vi "Add Array of New Shared Variables.vi"(7 "Data Type (Variant)":variant, 8 "error in":errorcluster, 9 "Variable Names":string[](array[string]), 10 "Library Path":path, 11 "Selected Library In":refnum<vi>) -> (0 "error out":errorcluster, 3 "Selected Library Out":refnum<vi>)   [LabVIEW 2017, in "Shared Variables Library.lvlib"]
doc: "Adds an array of shared variables, to the selected library."
uses:
  Shared Variables Library.lvlib
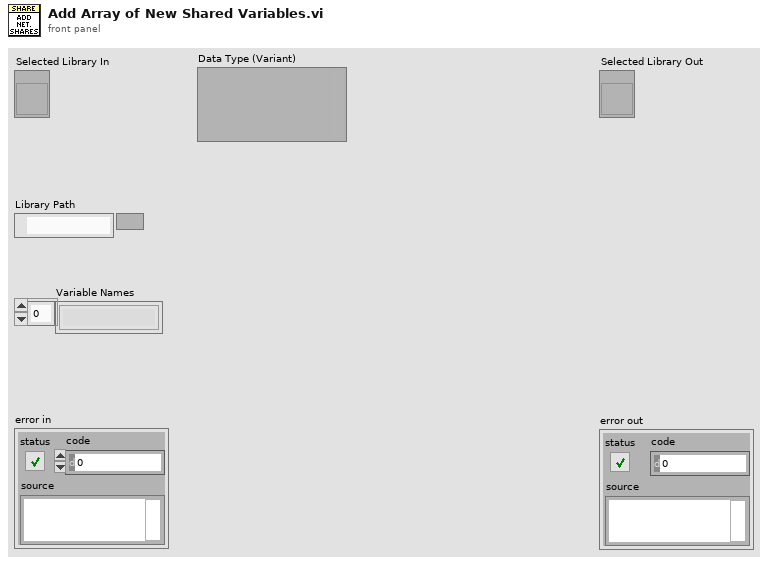
[diagram p1: front panel]
types:
  T1 = enum16{"Single-Process", "Network-Published", "Time-Triggered", "Industrial"}
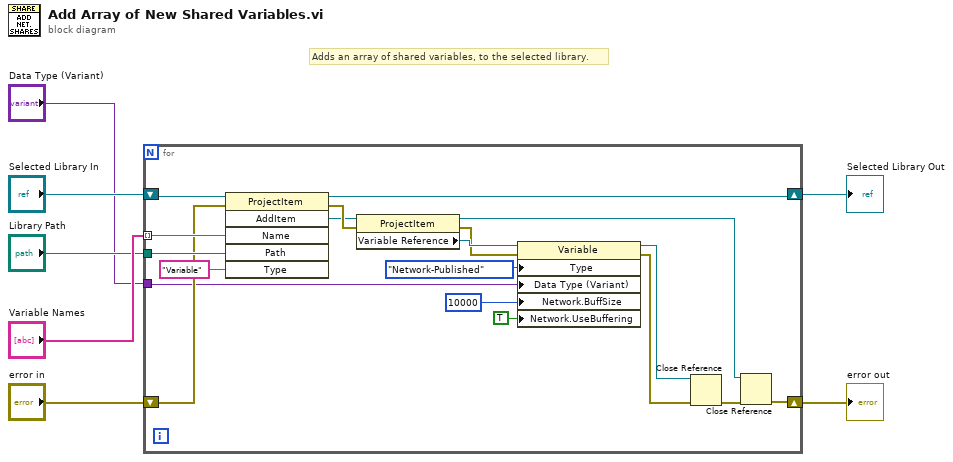
[diagram p0: block diagram]
diagram:
  # "Adds an array of shared variables, to the selected library."
  n1 = for {
    tunnel: "Variable Names" -> [w26] mode=indexing
    tunnel: "Library Path" -> [w23]
    shift-right: [w11] -> w3
    shift-left: "Selected Library In" -> [w24]
    shift-right: [w13] -> w2
    shift-left: "error in" -> [w19]
    tunnel: "Data Type (Variant)" -> [w10]
    n2 = invoke class="ProjectItem" method="AddItem"(reference=w24, error in=w19, "Name"=w26, "Path"=w23, "Type"="Variable") -> (reference out=w11:refnum<vi>, error out=w18:errorcluster, "AddItem"=w15:refnum<vi>)  [unwired: 1 in, 3 out]
    n3 = property class="ProjectItem"(reference=w15, error in=w18) -> (reference out=w12:refnum<vi>, error out=w17:errorcluster, "Variable Reference"=w22:refnum<vi>)
    n4 = property class="Variable"(reference=w22, error in=w17, "Type"=T1."Network-Published", "Data Type (Variant)"=w10, "Network.BuffSize"=u32 10000 ("Network:Buffer Size"), "Network.UseBuffering"=TRUE ("Network:Use Buffering")) -> (reference out=w20:refnum<vi>, error out=w16:errorcluster)
    n5 = Close Reference(reference=w20, error in (no error)=w16) -> (error out=w14:errorcluster)
    n6 = Close Reference(reference=w12, error in (no error)=w14) -> (error out=w13:errorcluster)
  }
  "Selected Library Out" <- w3
  "error out" <- w2
